vi "TestStand_Builder ( Split_Test_Group ).vi"(11 "Test_Case":string="\nPrecondition:\nPC_1. Wait.Sec(Delay=2)\n\nTestProcedure:\nTP_1. Wait.mSec(Delay=1000)  //Waits for ms\n\nReset:\nRST_1. Wait.Sec(Delay=2)  //Waits for sec\r\n") -> (1 "Reset":string[](array[string]), 2 "TestProcedure":string[](array[string]), 3 "Preconditions":string[](array[string]))   [LabVIEW 2018, in "TestStand_Control.lvlib"]
uses:
  TestStand_Control.lvlib
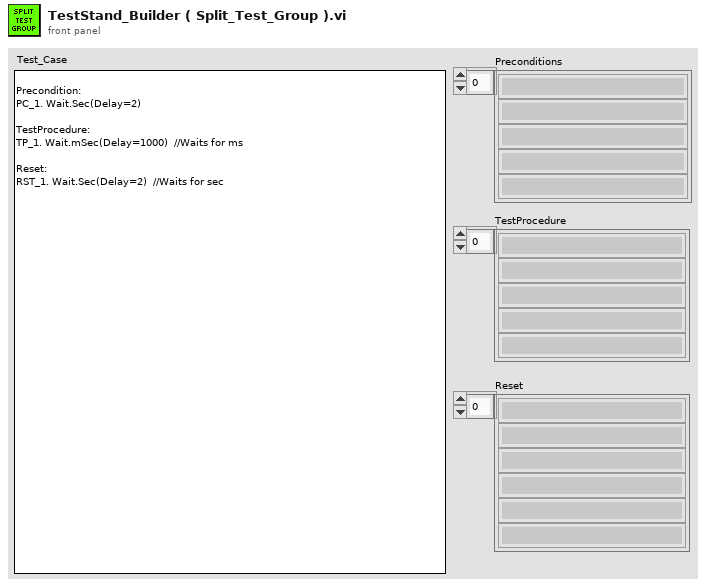
[diagram p1: front panel]
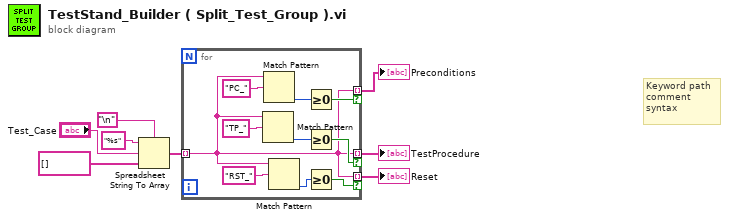
[diagram p0: block diagram]
diagram:
  # "Keyword path\ncomment\nsyntax"
  n1 = Spreadsheet String To Array(delimiter (Tab)="\n", format string="%s", spreadsheet string="Test_Case", array type (2D Dbl)=string[] []) -> (array=w4:string[])
  n2 = for {
    tunnel: w4 -> [w9] mode=indexing
    tunnel: [w9] -> w3 mode=indexing if=w16
    tunnel: [w9] -> w2 mode=indexing if=w13
    tunnel: [w9] -> w1 mode=indexing if=w10
    n3 = Match Pattern(string=w9, regular expression="TP_") -> (offset past match=w15:i32)  [unwired: 1 in, 3 out]
    n4 = Match Pattern(string=w9, regular expression="PC_") -> (offset past match=w17:i32)  [unwired: 1 in, 3 out]
    n5 = Match Pattern(string=w9, regular expression="RST_") -> (offset past match=w11:i32)  [unwired: 1 in, 3 out]
    n6 = Greater Or Equal To 0?(x=w17) -> (x >= 0?=w16:bool)
    n7 = Greater Or Equal To 0?(x=w15) -> (x >= 0?=w13:bool)
    n8 = Greater Or Equal To 0?(x=w11) -> (x >= 0?=w10:bool)
  }
  "Preconditions" <- w3
  "TestProcedure" <- w2
  "Reset" <- w1
